vi "loadDataToBuffer.vi"(8 "error in (no error)":errorcluster, 11 "niDAQmxAO in":refnum<class "niDAQmxAO.lvclass">) -> (0 "error out":errorcluster, 3 "niDAQmxAO out":refnum<class "niDAQmxAO.lvclass">)   [LabVIEW 2011, in "Hardware.lvlib" / "Channels.lvlib" / "niDAQmxAO.lvclass"]
uses:
  niDAQmxAO.lvclass
  <vilib>/DAQmx/write.llb/DAQmx Write (Analog 2D DBL NChan NSamp).vi
  <vilib>/DAQmx/miscellaneous.llb/DAQmx Fill In Error Info.vi
  AnalogOutput.lvclass
panel:
  out "Data":dbl[][](array[numeric])
  out "number of samples written per channel":u32
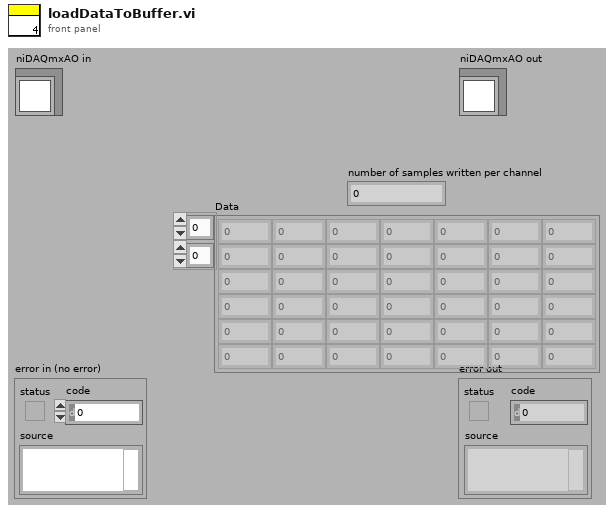
[diagram p1: front panel]
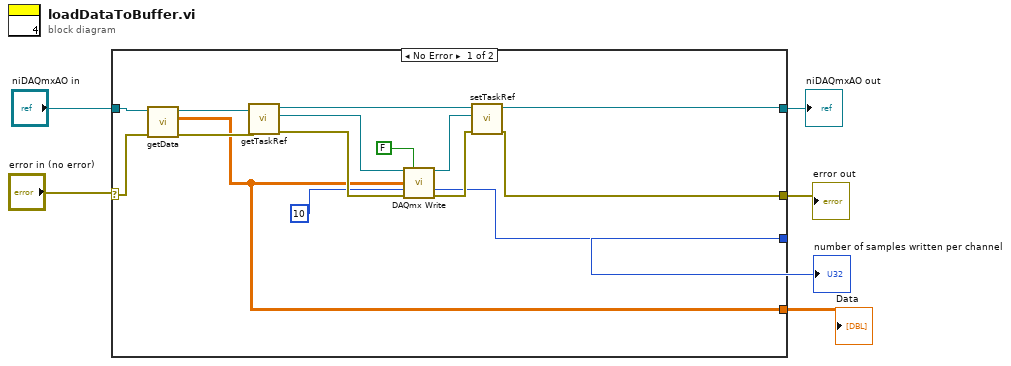
[diagram p0: block diagram]
diagram:
  n1 = case shown="No Error" "error in (no error)" {
    selector: "error in (no error)" -> [w20 w23]
    tunnel: [w8 w23] -> w5
    tunnel: [w14 w22] -> w3
    tunnel: "niDAQmxAO in" -> [w21 w22]
    tunnel: [w12 _] -> w2
    tunnel: [w10 _] -> w1
    frame No Error {
      n2 = call "getData.vi"("error in (no error)"=w20, "AnalogOutput.lvclass in"=w21) -> ("error out"=w18:errorcluster, "Data"=w10:dbl[][], "AnalogOutput.lvclass out"=w19:refnum<class "niDAQmxAO.lvclass">)  [unwired: 7 in]
      n3 = call "getTaskRef.vi"("error in (no error)"=w18, "niDAQmxAO.lvclass in"=w19) -> ("error out"=w17:errorcluster, "DAQmx Task Ref"=w9:refnum<k21>, "niDAQmxAO.lvclass out"=w16:refnum<class "niDAQmxAO.lvclass">)  [unwired: 7 in]
      n4 = call-poly <vilib>:"DAQmx Write.vi"("task/channels in"=w9, "auto start"=FALSE, "data"=w10, "timeout"=10, "error in"=w17) -> ("task out"=w7:refnum<k21>, "number of samples written per channel"=w12:u32, "error out"=w15:errorcluster)  [unwired: 8 in]
      n5 = call "setTaskRef.vi"("error in (no error)"=w15, "DAQmx Task Ref"=w7, "niDAQmxAO.lvclass in"=w16) -> ("error out"=w8:errorcluster, "niDAQmxAO.lvclass out"=w14:refnum<class "niDAQmxAO.lvclass">)  [unwired: 7 in]
    }
    frame Error {
    }
  }
  "error out" <- w5
  "niDAQmxAO out" <- w3
  "number of samples written per channel" <- w2
  "Data" <- w1
